vi "AudioTest.Unload SoundCheck Sequences.vi"(7 "Config":T1={"SeqDir"=path "C:/MTE/Audio Test/Config/SoundCheck/Sequences", "SoundCheckApp"=path "C:/SoundCheck 16.0-x64/SoundCheck 16.0 (x64).exe", "IP"="localhost", "Port"=4444, "Process Name"="SoundCheck 16.0 (x64)", "DataDir"=path "C:/MTE/Audio Test/Data/SoundCheck", "Window"=enum."Normal"}, 8 "error in":errorcluster, 9 "UUT Dir":path, 10 "Timeout(s)":dbl=60.0, 11 "Sequence":string="UTAH_EV2_SEQUENCE_20180820_DUMMY2.sqc") -> (0 "error out":errorcluster, 1 "App Launch Dur(s)":dbl, 2 "Duration":dbl, 3 "Ran to completion":bool)   [LabVIEW 2018]
uses:
  TypeDefs/SoundCheck Config.ctl
  Common/Utils/Errors/Error.Error Code List.ctl
  <vilib>/KATE/Files/File Utils.lvlib
  <vilib>/KATE/Time/Time Utils.lvlib
panel:
  out "Status":string
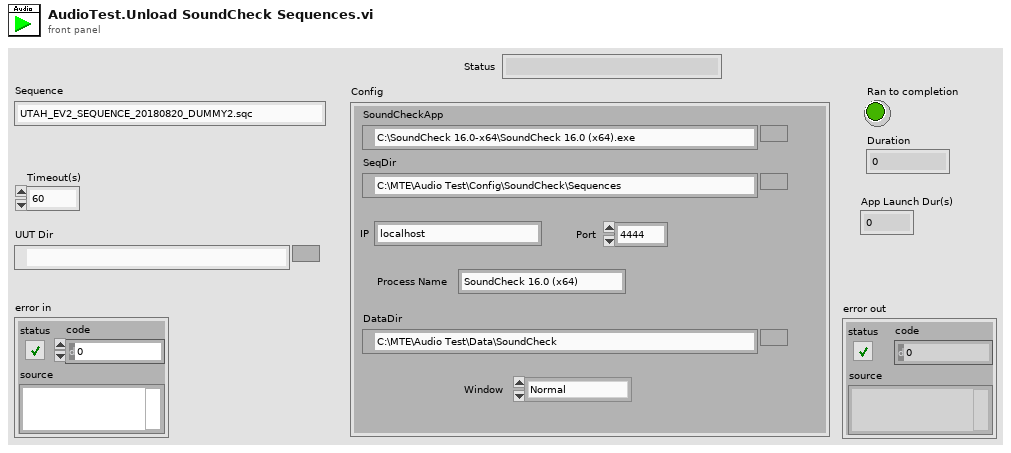
[diagram p1: front panel]
types:
  T1 = typedef "SoundCheck Config.ctl" = cluster{"SeqDir":path, "SoundCheckApp":path, "IP":string, "Port":u16, "Process Name":string, "DataDir":path, "Window":enum16{"Normal", "Minimized", "Hidden"}}
  T2 = typedef "Error.Error Code List.ctl" = i32
  T3 = cluster{"Config":T1, "Sequence":string, "Timeout(s)":dbl, "UUT Dir":path}
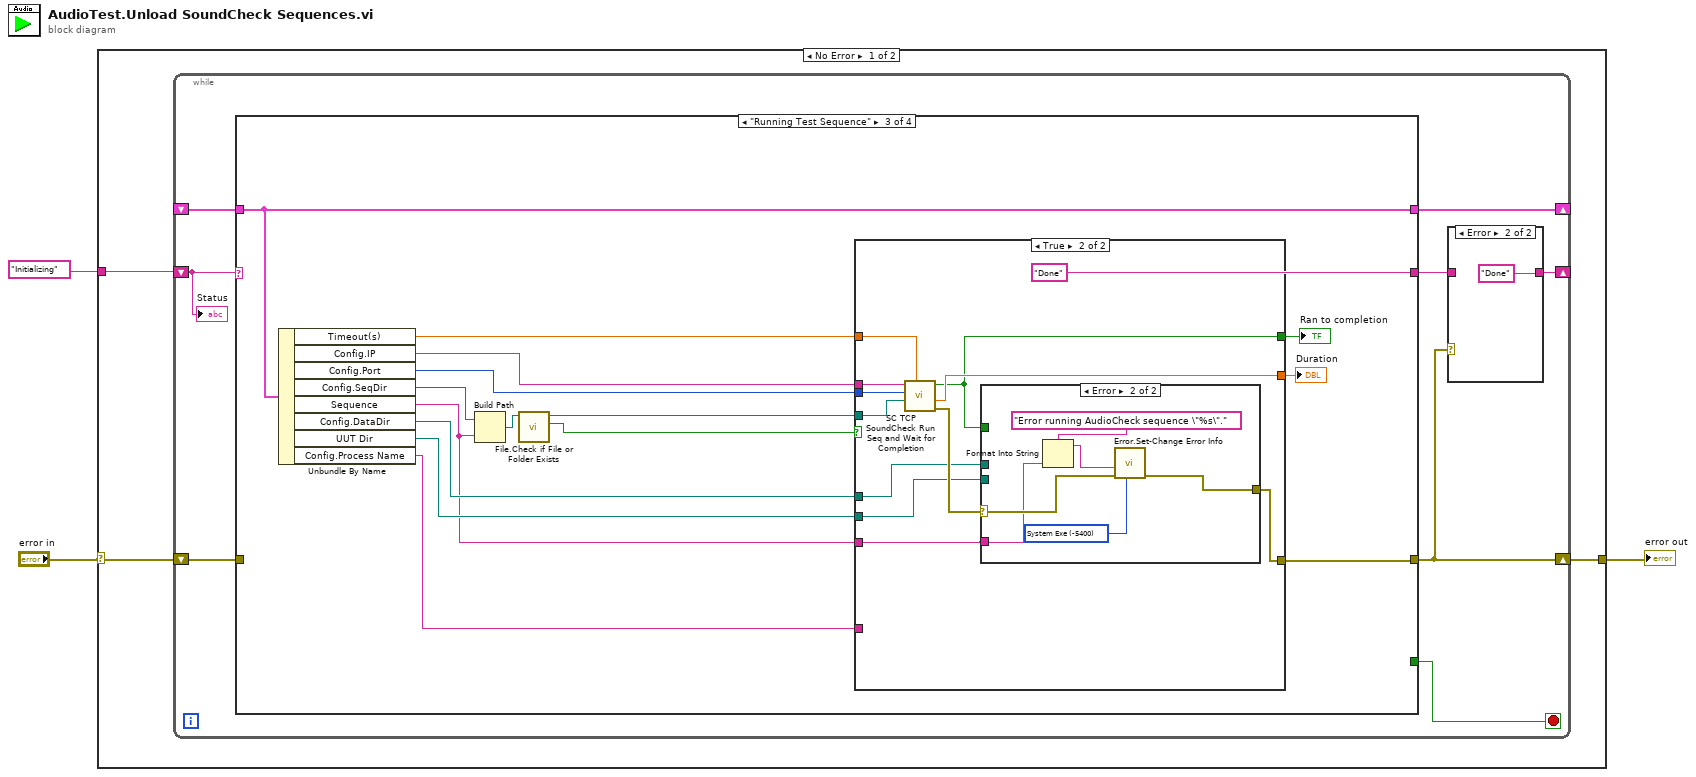
[diagram p0: block diagram]
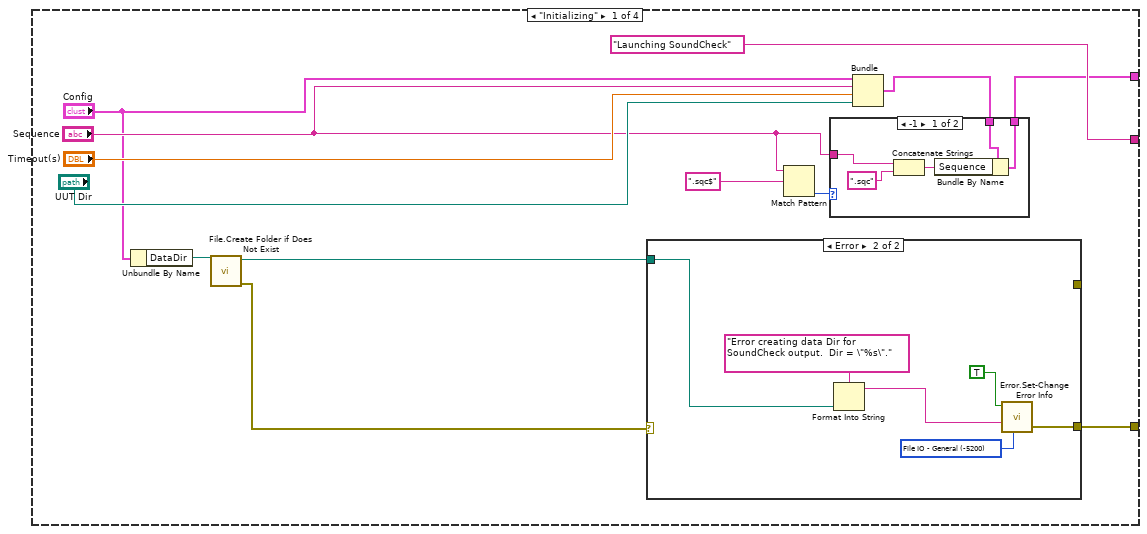
[diagram p3: hidden frame]
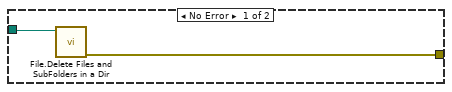
[diagram p5: hidden frame]
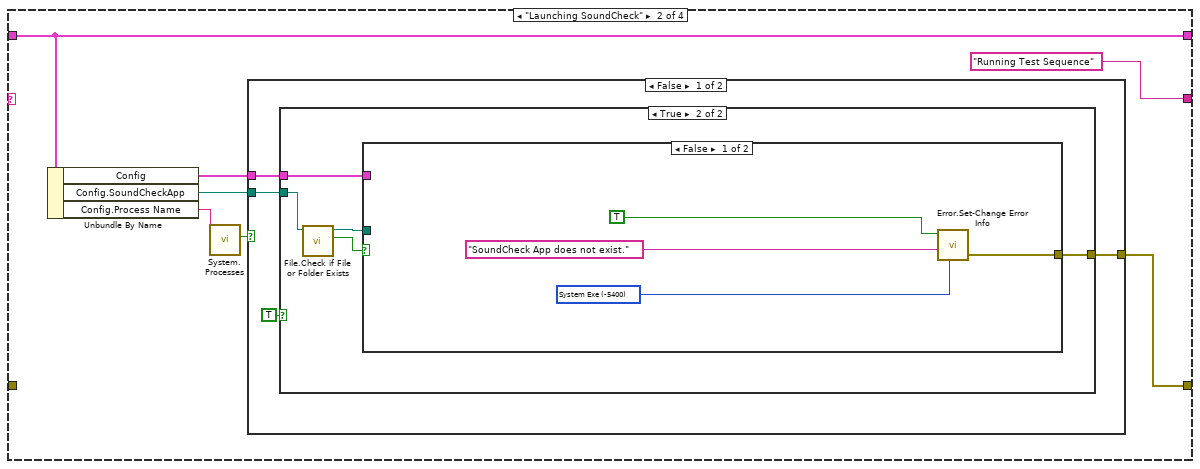
[diagram p6: hidden frame]
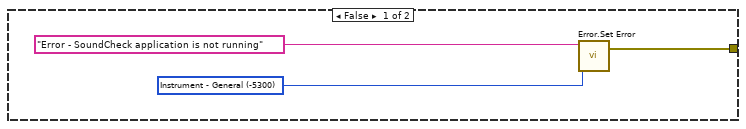
[diagram p7: hidden frame]
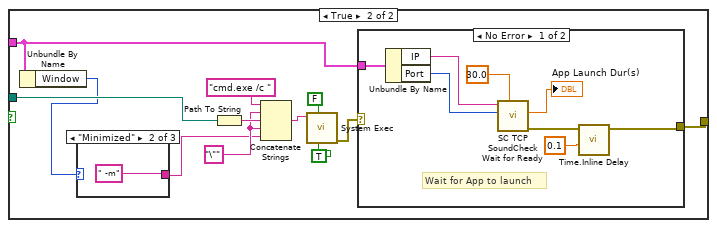
[diagram p8: hidden frame]
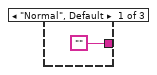
[diagram p9: hidden frame]
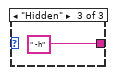
[diagram p10: hidden frame]
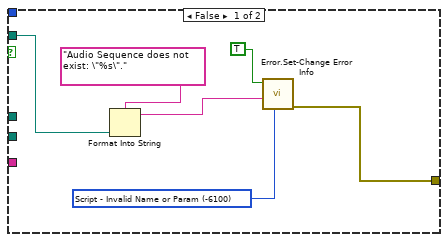
[diagram p13: hidden frame]
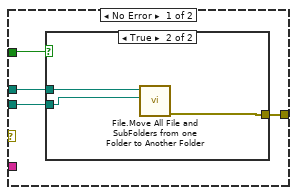
[diagram p14: hidden frame]
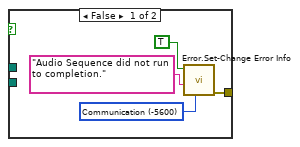
[diagram p15: hidden frame]
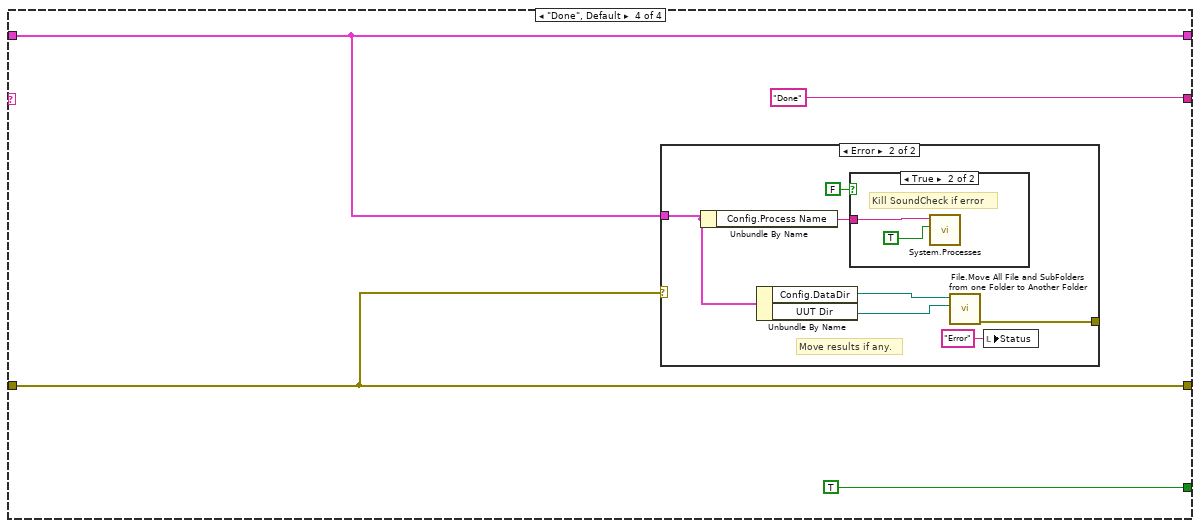
[diagram p16: hidden frame]
diagram:
  n1 = case shown="No Error" "error in" {
    selector: "error in" -> [w5 w154]
    tunnel: [w6 w154] -> w3
    tunnel: "Initializing" -> [w4 _]
    frame No Error {
      n2 = while {
        shift-right: [w14] -> _
        shift-left: _ -> [w13]
        shift-right: [w10] -> w6
        shift-left: w5 -> [w12]
        shift-right: [w8] -> _
        shift-left: w4 -> [w7]
        stop <- w11 stop-if-true
        n3 = case shown="\"Running Test Sequence\"" w7 {
          tunnel: [w19 w48 w105 w142] -> w14
          tunnel: w13 -> [_ w48 w105 w142]
          tunnel: ["Launching SoundCheck" "Running Test Sequence" "Done" "Done"] -> w9
          tunnel: w12 -> [_ _ _ w141]
          tunnel: [w24 w49 w97 w141] -> w10
          tunnel: [_ _ _ TRUE] -> w11
          frame "Initializing" {
            n4 = Unbundle By Name("Config") -> ("DataDir"=w26:path)
            n5 = call <vilib>:"File.Create Folder if Does Not Exist.vi"("Path"=w26) -> ("error out"=w25:errorcluster, "Dup Path"=w18:path)  [unwired: 8 in, 1 out]
            n6 = case shown="Error" w25 {
              tunnel: [_ w41] -> w24
              tunnel: w18 -> [w37 w39]
              tunnel: [w36 _] -> _
              frame No Error {
                n7 = call <vilib>:"File.Delete Files and SubFolders in a Dir.vi"("Dir"=w37) -> ("error out"=w36:errorcluster)  [unwired: 9 in, 1 out]
              }
              frame Error {
                w43 = T2 -5200 items=["No Error"=0, "Abort"=-2, "Misc"=-5000, "Fixture Error"=-5100, "File IO - General"=-5200, "FIle IO - Config Error"=-5201, "Instrument - General"=-5300, "Instrument - Serial Com"=-5301, "Instrument - Camera"=-5302, "Instrument - PS"=-5303, "Instrument - Oscilloscope"=-5304, "Instrument - Function Gen"=-5305, "Instrument - Load"=-5306, "Instrument - Meter"=-5307, "Instrument - Power Control"=-5308, "Instrument - Motion"=-5309, "Instrument - RF"=-5310, "System Exe"=-5400, "Image Processing"=-5500, "Communication"=-5600, "Script - Syntax Error"=-6000, "Script - Invalid Name or Param"=-6100, "Script - Timeout"=-6200, "Invalid Data"=-6300, "FW Update Error"=-6500] ("Std Code")
                n8 = Format Into String(format string="Error creating data Dir for SoundCheck output.  Dir = \"%s\"." ("Description"), w39) -> (resulting string=w38:string)  [unwired: 2 in, 1 out]
                n9 = call "Error.Set-Change Error Info.vi"("Std Code"=w43, "Description"=w38, "Set Error"=TRUE) -> ("error out"=w41:errorcluster)  [unwired: 8 in]
              }
            }
            n10 = Match Pattern(string="Sequence", regular expression=".sqc$") -> (offset past match=w22:i32)  [unwired: 1 in, 3 out]
            n11 = Bundle("Config"="Config", "Sequence"="Sequence", "Timeout(s)"="Timeout(s)", "UUT Dir"="UUT Dir") -> (w20:T3)  [unwired: 1 in]
            n12 = case shown="-1" w22 {
              tunnel: "Sequence" -> [w31 _]
              tunnel: w20 -> [w34 w35]
              tunnel: [w33 w35] -> w19
              frame -1 {
                n13 = Concatenate Strings(w31, ".sqc") -> (w32:string)
                n14 = Bundle By Name(cluster=w34, "Sequence"=w32) -> (w33:T3)
              }
              frame 0, Default {
              }
            }
          }
          frame "Launching SoundCheck" {
            n15 = Unbundle By Name(w48) -> ("Config"=w44:T1, "Config.SoundCheckApp"=w46:path, "Config.Process Name"=w47:string)
            n16 = call "System.Processes.vi"("Process Name"=w47) -> ("Is Running"=w45:bool)  [unwired: 8 in, 2 out]
            n17 = case shown="False" w45 {
              tunnel: [w54 _] -> w49
              tunnel: w46 -> [w53 _]
              tunnel: w44 -> [w52 _]
              frame False {
                n18 = case shown="True" TRUE {
                  tunnel: [w55 w62] -> w54
                  tunnel: w53 -> [_ w61]
                  tunnel: w52 -> [_ w58]
                  frame False {
                    w56 = T2 -5300 items=["No Error"=0, "Abort"=-2, "Misc"=-5000, "Fixture Error"=-5100, "File IO - General"=-5200, "FIle IO - Config Error"=-5201, "Instrument - General"=-5300, "Instrument - Serial Com"=-5301, "Instrument - Camera"=-5302, "Instrument - PS"=-5303, "Instrument - Oscilloscope"=-5304, "Instrument - Function Gen"=-5305, "Instrument - Load"=-5306, "Instrument - Meter"=-5307, "Instrument - Power Control"=-5308, "Instrument - Motion"=-5309, "Instrument - RF"=-5310, "System Exe"=-5400, "Image Processing"=-5500, "Communication"=-5600, "Script - Syntax Error"=-6000, "Script - Invalid Name or Param"=-6100, "Script - Timeout"=-6200, "Invalid Data"=-6300, "FW Update Error"=-6500] ("Std Code")
                    n19 = call "Error.Set Error.vi"("Code"=w56, "Desc"="Error - SoundCheck application is not running") -> ("error out"=w55:errorcluster)  [unwired: 5 in]
                  }
                  frame True {
                    n20 = call <vilib>:"File.Check if File or Folder Exists.vi"("Path"=w61) -> ("Exists"=w59:bool, "Dup Path"=w60:path)  [unwired: 6 in, 3 out]
                    n21 = case shown="False" w59 {
                      tunnel: [w66 w78] -> w62
                      tunnel: w60 -> [_ w70]
                      tunnel: w58 -> [_ w77]
                      frame False {
                        w63 = T2 -5400 items=["No Error"=0, "Abort"=-2, "Misc"=-5000, "Fixture Error"=-5100, "File IO - General"=-5200, "FIle IO - Config Error"=-5201, "Instrument - General"=-5300, "Instrument - Serial Com"=-5301, "Instrument - Camera"=-5302, "Instrument - PS"=-5303, "Instrument - Oscilloscope"=-5304, "Instrument - Function Gen"=-5305, "Instrument - Load"=-5306, "Instrument - Meter"=-5307, "Instrument - Power Control"=-5308, "Instrument - Motion"=-5309, "Instrument - RF"=-5310, "System Exe"=-5400, "Image Processing"=-5500, "Communication"=-5600, "Script - Syntax Error"=-6000, "Script - Invalid Name or Param"=-6100, "Script - Timeout"=-6200, "Invalid Data"=-6300, "FW Update Error"=-6500] ("Std Code")
                        n22 = call "Error.Set-Change Error Info.vi"("Std Code"=w63, "Description"="SoundCheck App does not exist.", "Set Error"=TRUE) -> ("error out"=w66:errorcluster)  [unwired: 8 in]
                      }
                      frame True {
                        w71 = "\"" ("string")
                        n23 = Unbundle By Name(w77) -> ("Window"=w68:enum16{"Normal", "Minimized", "Hidden"})
                        n24 = case shown="\"Minimized\"" w68 {
                          tunnel: ["" " -m" " -h"] -> w69
                          frame "Normal", Default {
                          }
                          frame "Minimized" {
                          }
                          frame "Hidden" {
                          }
                        }
                        n25 = Path To String(path=w70) -> (string=w72:string)
                        n26 = Concatenate Strings("cmd.exe /c ", w71, w72, w71, w69) -> (w76:string)
                        n27 = call <vilib>:"System Exec.vi"("run minimized? (F)"=TRUE, "wait until completion? (T)"=FALSE, "command line"=w76) -> ("error out"=w67:errorcluster)  [unwired: 5 in, 3 out]
                        n28 = case shown="No Error" w67 {
                          selector: w67 -> [_ w90]
                          tunnel: [w84 w90] -> w78
                          tunnel: w77 -> [w89 _]
                          frame No Error {
                            # "Wait for App to launch"
                            n29 = Unbundle By Name(w89) -> ("IP"=w88:string, "Port"=w87:u16)
                            n30 = call "SC TCP SoundCheck Wait for Ready.vi"("TimeOut(s)"=30.0, "port (4444)"=w87, "SoundCheck IP Address (localhost)"=w88) -> ("error out"=w85:errorcluster, "Duration"=→"App Launch Dur(s)":dbl)  [unwired: 6 in, 1 out]
                            n31 = call <vilib>:"Time.Inline Delay.vi"("Wait(secs)"=0.1, "error in top"=w85) -> ("error out top"=w84:errorcluster)  [unwired: 8 in, 1 out]
                          }
                          frame Error {
                          }
                        }
                      }
                    }
                  }
                }
              }
              frame True {
                # "Do nothing\nAlready running"
              }
            }
          }
          frame "Running Test Sequence" {
            n32 = Unbundle By Name(w105) -> ("Timeout(s)"=w103:dbl, "Config.IP"=w104:string, "Config.Port"=w102:u16, "Config.SeqDir"=w101:path, "Sequence"=w91:string, "Config.DataDir"=w95:path, "UUT Dir"=w94:path, "Config.Process Name"=w92:string)
            n33 = Build Path(base path=w101, name or relative path=w91) -> (appended path=w100:path)
            n34 = call <vilib>:"File.Check if File or Folder Exists.vi"("Path"=w100) -> ("Exists"=w93:bool, "Dup Path"=w99:path)  [unwired: 6 in, 3 out]
            n35 = case shown="True" w93 {
              tunnel: w104 -> [_ w123]
              tunnel: w103 -> [_ w122]
              tunnel: w102 -> [_ w121]
              tunnel: w99 -> [w109 w120]
              tunnel: [_ w119] -> w98
              tunnel: [w111 w117] -> w97
              tunnel: [_ w116] -> w96
              tunnel: w95 -> [_ w115]
              tunnel: w94 -> [_ w114]
              tunnel: w92 -> [_ _]
              tunnel: w91 -> [_ w113]
              frame False {
                w112 = T2 -6100 items=["No Error"=0, "Abort"=-2, "Misc"=-5000, "Fixture Error"=-5100, "File IO - General"=-5200, "FIle IO - Config Error"=-5201, "Instrument - General"=-5300, "Instrument - Serial Com"=-5301, "Instrument - Camera"=-5302, "Instrument - PS"=-5303, "Instrument - Oscilloscope"=-5304, "Instrument - Function Gen"=-5305, "Instrument - Load"=-5306, "Instrument - Meter"=-5307, "Instrument - Power Control"=-5308, "Instrument - Motion"=-5309, "Instrument - RF"=-5310, "System Exe"=-5400, "Image Processing"=-5500, "Communication"=-5600, "Script - Syntax Error"=-6000, "Script - Invalid Name or Param"=-6100, "Script - Timeout"=-6200, "Invalid Data"=-6300, "FW Update Error"=-6500] ("Std Code")
                n36 = Format Into String(format string="Audio Sequence does not exist: \"%s\"." ("Description"), w109) -> (resulting string=w108:string)  [unwired: 2 in, 1 out]
                n37 = call "Error.Set-Change Error Info.vi"("Std Code"=w112, "Description"=w108, "Set Error"=TRUE) -> ("error out"=w111:errorcluster)  [unwired: 8 in]
              }
              frame True {
                n38 = call "SC TCP SoundCheck Run Seq and Wait for Completion.vi"("TimeOut(s)"=w122, "Sequence to run (full path)"=w120, "port (4444)"=w121, "SoundCheck IP Address (localhost)"=w123) -> ("error out"=w118:errorcluster, "Duration"=w119:dbl, "Ran to completion"=w116:bool)  [unwired: 5 in]
                n39 = case shown="Error" w118 {
                  selector: w118 -> [_ w140]
                  tunnel: [w126 w138] -> w117
                  tunnel: w116 -> [w127 _]
                  tunnel: w115 -> [w125 _]
                  tunnel: w114 -> [w124 _]
                  tunnel: w113 -> [_ w135]
                  frame No Error {
                    n40 = case shown="True" w127 {
                      tunnel: [w128 w132] -> w126
                      tunnel: w125 -> [_ w134]
                      tunnel: w124 -> [_ w133]
                      frame False {
                        w131 = T2 -5600 items=["No Error"=0, "Abort"=-2, "Misc"=-5000, "Fixture Error"=-5100, "File IO - General"=-5200, "FIle IO - Config Error"=-5201, "Instrument - General"=-5300, "Instrument - Serial Com"=-5301, "Instrument - Camera"=-5302, "Instrument - PS"=-5303, "Instrument - Oscilloscope"=-5304, "Instrument - Function Gen"=-5305, "Instrument - Load"=-5306, "Instrument - Meter"=-5307, "Instrument - Power Control"=-5308, "Instrument - Motion"=-5309, "Instrument - RF"=-5310, "System Exe"=-5400, "Image Processing"=-5500, "Communication"=-5600, "Script - Syntax Error"=-6000, "Script - Invalid Name or Param"=-6100, "Script - Timeout"=-6200, "Invalid Data"=-6300, "FW Update Error"=-6500] ("Std Code")
                        n41 = call "Error.Set-Change Error Info.vi"("Std Code"=w131, "Description"="Audio Sequence did not run to completion.", "Set Error"=TRUE) -> ("error out"=w128:errorcluster)  [unwired: 8 in]
                      }
                      frame True {
                        n42 = call "File.Move All File and SubFolders from one Folder to Another Folder.vi"("Destination Folder"=w133, "Source Folder"=w134) -> ("error out"=w132:errorcluster)  [unwired: 8 in, 1 out]
                      }
                    }
                  }
                  frame Error {
                    w139 = T2 -5400 items=["No Error"=0, "Abort"=-2, "Misc"=-5000, "Fixture Error"=-5100, "File IO - General"=-5200, "FIle IO - Config Error"=-5201, "Instrument - General"=-5300, "Instrument - Serial Com"=-5301, "Instrument - Camera"=-5302, "Instrument - PS"=-5303, "Instrument - Oscilloscope"=-5304, "Instrument - Function Gen"=-5305, "Instrument - Load"=-5306, "Instrument - Meter"=-5307, "Instrument - Power Control"=-5308, "Instrument - Motion"=-5309, "Instrument - RF"=-5310, "System Exe"=-5400, "Image Processing"=-5500, "Communication"=-5600, "Script - Syntax Error"=-6000, "Script - Invalid Name or Param"=-6100, "Script - Timeout"=-6200, "Invalid Data"=-6300, "FW Update Error"=-6500] ("Std Code")
                    n43 = Format Into String(format string="Error running AudioCheck sequence \"%s\"." ("Description"), w135) -> (resulting string=w136:string)  [unwired: 2 in, 1 out]
                    n44 = call "Error.Set-Change Error Info.vi"("Std Code"=w139, "error in"=w140, "Description"=w136) -> ("error out"=w138:errorcluster)  [unwired: 8 in]
                  }
                }
              }
            }
            "Duration" <- w98
            "Ran to completion" <- w96
          }
          frame "Done", Default {
            n45 = case shown="Error" w141 {
              tunnel: w142 -> [_ w147]
              tunnel: [_ w146] -> _
              frame No Error {
              }
              frame Error {
                # "Move results if any."
                n46 = Unbundle By Name(w147) -> ("Config.Process Name"=w151:string)
                n47 = Unbundle By Name(w147) -> ("Config.DataDir"=w148:path, "UUT Dir"=w149:path)
                n48 = case shown="True" FALSE {
                  tunnel: w151 -> [_ w153]
                  frame False {
                  }
                  frame True {
                    # "Kill SoundCheck if error"
                    n49 = call "System.Processes.vi"("Kill"=TRUE, "Process Name"=w153) -> ()  [unwired: 7 in, 3 out]
                  }
                }
                n50 = call "File.Move All File and SubFolders from one Folder to Another Folder.vi"("Destination Folder"=w149, "Source Folder"=w148) -> ("error out"=w146:errorcluster)  [unwired: 8 in, 1 out]
                n51 = local write "Status"("Error" ("Status")) -> ()
              }
            }
          }
        }
        n52 = case shown="Error" w10 {
          tunnel: w9 -> [w15 _]
          tunnel: [w15 "Done"] -> w8
          frame No Error {
          }
          frame Error {
          }
        }
        "Status" <- w7
      }
    }
    frame Error {
    }
  }
  "error out" <- w3
